vi "メイン.vi"() -> (2 "測定周期/ms":dbl, 3 "値転記用配列":T2[](array[typedef]))   [LabVIEW 2021] (continued)
                  tunnel: w3711 -> [w3725]
                  tunnel: [w3725] -> w3710
                  frame #0 {
                    w3720 = T9 {"Horizontal"=-51, "Vertical"=72} ("座標 2")
                    n1890 = control-ref of="このVI"() -> (w3724:refnum<vi>)
                    n1891 = property on="ペーン 2" class="Pane"("Origin"=w3720) -> ()  [unwired: 2 in, 2 out]
                    n1892 = property on="ペーン 2" class="Pane"("Origin"=w3720) -> ()  [unwired: 2 in, 2 out]
                    n1893 = control-ref of="このVI"() -> (w3722:refnum<vi>)
                    n1894 = Unbundle(w3720) -> ("Vertical"=w3723:i16)  [unwired: 1 out]
                    n1895 = Unbundle(w3720) -> ("Vertical"=w3721:i16)  [unwired: 1 out]
                    n1896 = call "メイン_装飾移動サブ.vi"("Y軸座標入力"=w3723, "VI入力"=w3724) -> ()  [unwired: 10 in]
                    n1897 = call "メイン_装飾枠移動サブ.vi"("Y軸座標入力"=w3721, "VI入力"=w3722) -> ()  [unwired: 10 in]
                  }
                }
              }
              frame #1 {
                w3955 = T8."Enabled" ("無効")
                # "⑪ボタンの無効解除"
                n1898 = local write "測定新値\nリセット用 2"(TRUE) -> ()
                n1899 = for {
                  N: 12 -> [_]
                  tunnel: w3955 -> [w3958]
                  i -> [w3959]
                  n1900 = case shown="11" w3959 {
                    tunnel: w3958 -> [w3960 w3961 w3962 w3963 w3964 w3965 w3966 w3967 w3968 w3969 w3970 w3971]
                    frame 0, Default {
                      n1901 = property on="メイン測定ボタン_単発 1" class="Bool (指定)"("DisabledEnum"=w3960) -> ()  [unwired: 2 in, 2 out]
                      n1902 = property on="メイン測定ボタン_連続 1" class="Bool (指定)"("DisabledEnum"=w3960) -> ()  [unwired: 2 in, 2 out]
                    }
                    frame 1 {
                      n1903 = property on="メイン測定ボタン_単発 2" class="Bool (指定)"("DisabledEnum"=w3961) -> ()  [unwired: 2 in, 2 out]
                      n1904 = property on="メイン測定ボタン_連続 2" class="Bool (指定)"("DisabledEnum"=w3961) -> ()  [unwired: 2 in, 2 out]
                    }
                    frame 2 {
                      n1905 = property on="メイン測定ボタン_単発 3" class="Bool (指定)"("DisabledEnum"=w3962) -> ()  [unwired: 2 in, 2 out]
                      n1906 = property on="メイン測定ボタン_連続 3" class="Bool (指定)"("DisabledEnum"=w3962) -> ()  [unwired: 2 in, 2 out]
                    }
                    frame 3 {
                      n1907 = property on="メイン測定ボタン_単発 4" class="Bool (指定)"("DisabledEnum"=w3963) -> ()  [unwired: 2 in, 2 out]
                      n1908 = property on="メイン測定ボタン_連続 4" class="Bool (指定)"("DisabledEnum"=w3963) -> ()  [unwired: 2 in, 2 out]
                    }
                    frame 4 {
                      n1909 = property on="メイン測定ボタン_単発 5" class="Bool (指定)"("DisabledEnum"=w3964) -> ()  [unwired: 2 in, 2 out]
                      n1910 = property on="メイン測定ボタン_連続 5" class="Bool (指定)"("DisabledEnum"=w3964) -> ()  [unwired: 2 in, 2 out]
                    }
                    frame 5 {
                      n1911 = property on="メイン測定ボタン_連続 6" class="Bool (指定)"("DisabledEnum"=w3965) -> ()  [unwired: 2 in, 2 out]
                      n1912 = property on="メイン測定ボタン_単発 6" class="Bool (指定)"("DisabledEnum"=w3965) -> ()  [unwired: 2 in, 2 out]
                    }
                    frame 6 {
                      n1913 = property on="メイン測定ボタン_連続 7" class="Bool (指定)"("DisabledEnum"=w3966) -> ()  [unwired: 2 in, 2 out]
                      n1914 = property on="メイン測定ボタン_単発 7" class="Bool (指定)"("DisabledEnum"=w3966) -> ()  [unwired: 2 in, 2 out]
                    }
                    frame 7 {
                      n1915 = property on="メイン測定ボタン_単発 8" class="Bool (指定)"("DisabledEnum"=w3967) -> ()  [unwired: 2 in, 2 out]
                      n1916 = property on="メイン測定ボタン_連続 8" class="Bool (指定)"("DisabledEnum"=w3967) -> ()  [unwired: 2 in, 2 out]
                    }
                    frame 8 {
                      n1917 = property on="メイン測定ボタン_単発 9" class="Bool (指定)"("DisabledEnum"=w3968) -> ()  [unwired: 2 in, 2 out]
                      n1918 = property on="メイン測定ボタン_連続 9" class="Bool (指定)"("DisabledEnum"=w3968) -> ()  [unwired: 2 in, 2 out]
                    }
                    frame 9 {
                      n1919 = property on="メイン測定ボタン_単発 10" class="Bool (指定)"("DisabledEnum"=w3969) -> ()  [unwired: 2 in, 2 out]
                      n1920 = property on="メイン測定ボタン_連続 10" class="Bool (指定)"("DisabledEnum"=w3969) -> ()  [unwired: 2 in, 2 out]
                    }
                    frame 10 {
                      n1921 = property on="メイン測定ボタン_単発 11" class="Bool (指定)"("DisabledEnum"=w3970) -> ()  [unwired: 2 in, 2 out]
                      n1922 = property on="メイン測定ボタン_連続 11" class="Bool (指定)"("DisabledEnum"=w3970) -> ()  [unwired: 2 in, 2 out]
                    }
                    frame 11 {
                      n1923 = property on="メイン測定ボタン_連続 12" class="Bool (指定)"("DisabledEnum"=w3971) -> ()  [unwired: 2 in, 2 out]
                      n1924 = property on="メイン測定ボタン_単発 12" class="Bool (指定)"("DisabledEnum"=w3971) -> ()  [unwired: 2 in, 2 out]
                    }
                  }
                }
                n1925 = property on="TOPページへ" class="Bool"("DisabledEnum"=w3955) -> ()  [unwired: 2 in, 2 out]
                n1926 = property on="保存して終了" class="Bool"("DisabledEnum"=w3955) -> ()  [unwired: 2 in, 2 out]
                n1927 = property on="保存せずに" class="Bool"("DisabledEnum"=w3955) -> ()  [unwired: 2 in, 2 out]
              }
            }
          }
          frame True {
          }
        }
      }
      frame "測定3" {
        # "⑦"
        # "項目別のボタンで測定を行う為、項目分必要"
        n1928 = local read "測定旧値 3"() -> (w3975:bool)
        n1929 = case shown="FALSE" w3975 {
          tunnel: w3973 -> [w3978 w4241]
          tunnel: [w3977 w4241] -> w3974
          frame False {
            n1930 = flat-sequence {
              tunnel: w3978 -> [w3988]
              tunnel: [w3980] -> w3976
              tunnel: [w4226] -> w3977
              tunnel: w3976 -> [w4226]
              frame #0 {
                # "※複製コピー時変更する項目\n①②\nローカル変数\n\n入れ子のケースストラクチャ\"2\"を複製\n\n0～数だけ変更する\n③④⑤\nローカル変数\n\n※AB\n行番号の変更をする必要がある\n\n--------------------------------\nこの後イベントストラクチャ複製する\n--------------------------------\nイベントストラクチャ複製後\n\n⑦⑧\nローカル変数\n⑨\n装飾体の位置設定\n-51は固定\n前ケースの数値+72\n⑩\n測定新値リセット用\nのボタンが複製されているので、\nフロントパネルを整理する\n⑪\nプロパティノード\nボタンの無効解除クリア以外全てのボタン対象"
                # "実測完了の簡易疑似コード\n\n1)測定モードが単発・連続、多点かで転記する配列を変える\n2)値転記用配列へ転記\n\nここからゲージ分を繰り返す必要がある\n\n3)配列0を取り出す\n4)配列0のポートNoを取り出す\n5)メイン測定_設定配列(測定1の対象配列)のポートNoと比較\n6)同じだったら処理をする。違ったら何もしない\n7)同じだったら配列0のメインON/OFF_設定1の使用ON/OFFがTrueかFalseか\nFlaseだったら前回値転記用配列から前回の値をメイン設定_設定へ転記\nTrueだったらメイン設定_設定の測定モードから\n0単発、1連続、3多点\nの処理を行う\n8)測定値をメイン設定_設定へ転記したら、前回転記用配列へ転記する"
                # "⑨"
                # "⑧"
                # "②"
                # "グループNO(表示上はポートNo)が同じだったら値を転記する\n\n測定した配列のグループNOと値転記用配列の他の指標グループNOを比較する\n＝だったら、対象の配列のON/OFFボタンがTrueか確認し、\nTrueだったら、測定モードによって、値かMAX、MINの数値を転記する\n\nグループNOが同じでなければ、転記しない(何もしない)"
                # "まず値転記用配列に測定の値を転記"
                # "実測定画面vi動作"
                n1931 = local read "メイン設定_設定 3"() -> (w3983:T2)
                n1932 = local read "測定新値 3"() -> (→"測定新値\nリセット用 3":bool)
                n1933 = local read "測定周期/ms"() -> (w3981:dbl)
                n1934 = Unbundle By Name(w3983) -> ("測定モード"=w3984:u16)
                n1935 = call "実測定画面.vi"("実測設定項目配列_\nメインからの転記"=w3988, "測定周期/ms_制御器"=w3981) -> ("実測設定項目配列_\nゲージIOへ転記用"=w3986:T2[], "実測設定項目配列_\n多点測定メイン転記用"=w3985:T2[])  [unwired: 11 in, 1 out]
                n1936 = case shown="1" w3984 {
                  tunnel: w3986 -> [w3995 w3996 _]
                  tunnel: [w3995 w3996 w3997] -> w3979
                  tunnel: w3985 -> [_ _ w3997]
                  frame 0, Default {
                  }
                  frame 1 {
                  }
                  frame 2 {
                  }
                }
                n1937 = for {
                  N: 32 -> [_]
                  tunnel: w3979 -> [w4004]
                  i -> [w3999]
                  # "①"
                  # "※複製コピーはこのケースで行う"
                  # "32回分"
                  # "比較する固定GNO"
                  n1938 = local read "メイン設定_設定 3"() -> (w3998:T2)
                  n1939 = Index Array(array=w4004, index=w3999) -> (element=w4003:T2)
                  n1940 = Unbundle By Name(w3998) -> ("ポートNo."=w4002:dbl)
                  n1941 = Unbundle By Name(w4003) -> ("ポートNo."=w4001:dbl)
                  n1942 = Equal?(x=w4002, y=w4001) -> (x = y?=w4000:bool)
                  n1943 = case shown="TRUE" w4000 {
                    tunnel: w4003 -> [_ w4006]
                    tunnel: w3999 -> [_ w4005]
                    frame False {
                    }
                    frame True {
                      n1944 = case shown="0, デフォルト" w4005 {
                        tunnel: w4006 -> [w4022 w4040 w4058 w4076 w4094 w4112 w4130 w4148 w4166 w4184 w4202 w4220]
                        tunnel: w4005 -> [w4021 w4039 w4057 w4075 w4093 w4111 w4129 w4147 w4165 w4183 w4201 w4219]
                        frame 0, Default {
                          w4012 = 2
                          # "B"
                          # "A"
                          # "csv作成の為表へクラスタ(実測値)書き込み"
                          # "⑤"
                          # "③"
                          # "④"
                          n1945 = local read "メインON/OFF_\n設定 1"() -> (w4023:T1)
                          n1946 = Unbundle By Name(w4023) -> ("使用ON/OFF"=w4019:bool)
                          n1947 = control-ref of="前回値転記用配列"() -> (w4017:refnum<vi>)
                          n1948 = local read "メイン設定_設定 1"() -> (w4024:T2)
                          n1949 = call "メイン_測定値配列_CSV転記サブ.vi"("メイン設定_設定入力"=w4024, "ループ反復数値入力"=w4021, "実測設定項目"=w4022, "使用ON/OFF"=w4019, "前回値転記用配列"=w4017) -> ("ループ反復数値出力"=w4020:i32, "メイン設定_設定出力"=w4018:T2)  [unwired: 5 in]
                          n1950 = local write "メイン設定_設定 1"(w4018) -> ()
                          n1951 = Add(x=2, y=w4020) -> (x+y=w4013:i32)
                          n1952 = Add(x=w4020, y=3) -> (x+y=w4011:i32)
                          n1953 = local read "csv作成表"() -> (w4007:string[][])
                          n1954 = Unbundle By Name(w4018) -> ("実測値(MAX)"=w4014:string, "実測値(MIN)"=w4015:string)
                          n1955 = Replace Array Subset(array=w4007, new element #1=w4014, index (row) #1=w4012, index (col) #1=w4013, new element #2=w4015, index (row) #2=w4012, index (col) #2=w4011) -> (w4009:string[][])
                          n1956 = Select(t=w4009, s=w4019, f=w4007) -> (s? t:f=w4010:string[][])
                          n1957 = local write "csv作成表"(w4010) -> ()
                        }
                        frame 1 {
                          w4030 = 2
                          # "B"
                          # "A"
                          # "csv作成の為表へクラスタ(実測値)書き込み"
                          # "⑤"
                          # "③"
                          # "④"
                          n1958 = local read "メインON/OFF_\n設定 2"() -> (w4041:T1)
                          n1959 = Unbundle By Name(w4041) -> ("使用ON/OFF"=w4037:bool)
                          n1960 = control-ref of="前回値転記用配列"() -> (w4035:refnum<vi>)
                          n1961 = local read "メイン設定_設定 2"() -> (w4042:T2)
                          n1962 = call "メイン_測定値配列_CSV転記サブ.vi"("メイン設定_設定入力"=w4042, "ループ反復数値入力"=w4039, "実測設定項目"=w4040, "使用ON/OFF"=w4037, "前回値転記用配列"=w4035) -> ("ループ反復数値出力"=w4038:i32, "メイン設定_設定出力"=w4036:T2)  [unwired: 5 in]
                          n1963 = local write "メイン設定_設定 2"(w4036) -> ()
                          n1964 = Add(x=3, y=w4038) -> (x+y=w4031:i32)
                          n1965 = Add(x=w4038, y=4) -> (x+y=w4029:i32)
                          n1966 = local read "csv作成表"() -> (w4025:string[][])
                          n1967 = Unbundle By Name(w4036) -> ("実測値(MAX)"=w4032:string, "実測値(MIN)"=w4033:string)
                          n1968 = Replace Array Subset(array=w4025, new element #1=w4032, index (row) #1=w4030, index (col) #1=w4031, new element #2=w4033, index (row) #2=w4030, index (col) #2=w4029) -> (w4027:string[][])
                          n1969 = Select(t=w4027, s=w4037, f=w4025) -> (s? t:f=w4028:string[][])
                          n1970 = local write "csv作成表"(w4028) -> ()
                        }
                        frame 2 {
                          w4048 = 2
                          # "B"
                          # "A"
                          # "csv作成の為表へクラスタ(実測値)書き込み"
                          # "⑤"
                          # "③"
                          # "④"
                          n1971 = local read "メインON/OFF_\n設定 3"() -> (w4059:T1)
                          n1972 = Unbundle By Name(w4059) -> ("使用ON/OFF"=w4055:bool)
                          n1973 = control-ref of="前回値転記用配列"() -> (w4053:refnum<vi>)
                          n1974 = local read "メイン設定_設定 3"() -> (w4060:T2)
                          n1975 = call "メイン_測定値配列_CSV転記サブ.vi"("メイン設定_設定入力"=w4060, "ループ反復数値入力"=w4057, "実測設定項目"=w4058, "使用ON/OFF"=w4055, "前回値転記用配列"=w4053) -> ("ループ反復数値出力"=w4056:i32, "メイン設定_設定出力"=w4054:T2)  [unwired: 5 in]
                          n1976 = local write "メイン設定_設定 3"(w4054) -> ()
                          n1977 = Add(x=4, y=w4056) -> (x+y=w4049:i32)
                          n1978 = Add(x=w4056, y=5) -> (x+y=w4047:i32)
                          n1979 = local read "csv作成表"() -> (w4043:string[][])
                          n1980 = Unbundle By Name(w4054) -> ("実測値(MAX)"=w4050:string, "実測値(MIN)"=w4051:string)
                          n1981 = Replace Array Subset(array=w4043, new element #1=w4050, index (row) #1=w4048, index (col) #1=w4049, new element #2=w4051, index (row) #2=w4048, index (col) #2=w4047) -> (w4045:string[][])
                          n1982 = Select(t=w4045, s=w4055, f=w4043) -> (s? t:f=w4046:string[][])
                          n1983 = local write "csv作成表"(w4046) -> ()
                        }
                        frame 3 {
                          w4066 = 2
                          # "B"
                          # "A"
                          # "csv作成の為表へクラスタ(実測値)書き込み"
                          # "⑤"
                          # "③"
                          # "④"
                          n1984 = local read "メインON/OFF_\n設定 4"() -> (w4077:T1)
                          n1985 = Unbundle By Name(w4077) -> ("使用ON/OFF"=w4073:bool)
                          n1986 = control-ref of="前回値転記用配列"() -> (w4071:refnum<vi>)
                          n1987 = local read "メイン設定_設定 4"() -> (w4078:T2)
                          n1988 = call "メイン_測定値配列_CSV転記サブ.vi"("メイン設定_設定入力"=w4078, "ループ反復数値入力"=w4075, "実測設定項目"=w4076, "使用ON/OFF"=w4073, "前回値転記用配列"=w4071) -> ("ループ反復数値出力"=w4074:i32, "メイン設定_設定出力"=w4072:T2)  [unwired: 5 in]
                          n1989 = local write "メイン設定_設定 4"(w4072) -> ()
                          n1990 = Add(x=5, y=w4074) -> (x+y=w4067:i32)
                          n1991 = Add(x=w4074, y=6) -> (x+y=w4065:i32)
                          n1992 = local read "csv作成表"() -> (w4061:string[][])
                          n1993 = Unbundle By Name(w4072) -> ("実測値(MAX)"=w4068:string, "実測値(MIN)"=w4069:string)
                          n1994 = Replace Array Subset(array=w4061, new element #1=w4068, index (row) #1=w4066, index (col) #1=w4067, new element #2=w4069, index (row) #2=w4066, index (col) #2=w4065) -> (w4063:string[][])
                          n1995 = Select(t=w4063, s=w4073, f=w4061) -> (s? t:f=w4064:string[][])
                          n1996 = local write "csv作成表"(w4064) -> ()
                        }
                        frame 4 {
                          w4084 = 2
                          # "B"
                          # "A"
                          # "csv作成の為表へクラスタ(実測値)書き込み"
                          # "⑤"
                          # "③"
                          # "④"
                          n1997 = local read "メインON/OFF_\n設定 5"() -> (w4095:T1)
                          n1998 = Unbundle By Name(w4095) -> ("使用ON/OFF"=w4091:bool)
                          n1999 = control-ref of="前回値転記用配列"() -> (w4089:refnum<vi>)
                          n2000 = local read "メイン設定_設定 5"() -> (w4096:T2)
                          n2001 = call "メイン_測定値配列_CSV転記サブ.vi"("メイン設定_設定入力"=w4096, "ループ反復数値入力"=w4093, "実測設定項目"=w4094, "使用ON/OFF"=w4091, "前回値転記用配列"=w4089) -> ("ループ反復数値出力"=w4092:i32, "メイン設定_設定出力"=w4090:T2)  [unwired: 5 in]
                          n2002 = local write "メイン設定_設定 5"(w4090) -> ()
                          n2003 = Add(x=6, y=w4092) -> (x+y=w4085:i32)
                          n2004 = Add(x=w4092, y=7) -> (x+y=w4083:i32)
                          n2005 = local read "csv作成表"() -> (w4079:string[][])
                          n2006 = Unbundle By Name(w4090) -> ("実測値(MAX)"=w4086:string, "実測値(MIN)"=w4087:string)
                          n2007 = Replace Array Subset(array=w4079, new element #1=w4086, index (row) #1=w4084, index (col) #1=w4085, new element #2=w4087, index (row) #2=w4084, index (col) #2=w4083) -> (w4081:string[][])
                          n2008 = Select(t=w4081, s=w4091, f=w4079) -> (s? t:f=w4082:string[][])
                          n2009 = local write "csv作成表"(w4082) -> ()
                        }
                        frame 5 {
                          w4102 = 2
                          # "B"
                          # "A"
                          # "csv作成の為表へクラスタ(実測値)書き込み"
                          # "⑤"
                          # "③"
                          # "④"
                          n2010 = local read "メインON/OFF_\n設定 6"() -> (w4113:T1)
                          n2011 = Unbundle By Name(w4113) -> ("使用ON/OFF"=w4109:bool)
                          n2012 = control-ref of="前回値転記用配列"() -> (w4107:refnum<vi>)
                          n2013 = local read "メイン設定_設定 6"() -> (w4114:T2)
                          n2014 = call "メイン_測定値配列_CSV転記サブ.vi"("メイン設定_設定入力"=w4114, "ループ反復数値入力"=w4111, "実測設定項目"=w4112, "使用ON/OFF"=w4109, "前回値転記用配列"=w4107) -> ("ループ反復数値出力"=w4110:i32, "メイン設定_設定出力"=w4108:T2)  [unwired: 5 in]
                          n2015 = local write "メイン設定_設定 6"(w4108) -> ()
                          n2016 = Add(x=7, y=w4110) -> (x+y=w4103:i32)
                          n2017 = Add(x=w4110, y=8) -> (x+y=w4101:i32)
                          n2018 = local read "csv作成表"() -> (w4097:string[][])
                          n2019 = Unbundle By Name(w4108) -> ("実測値(MAX)"=w4104:string, "実測値(MIN)"=w4105:string)
                          n2020 = Replace Array Subset(array=w4097, new element #1=w4104, index (row) #1=w4102, index (col) #1=w4103, new element #2=w4105, index (row) #2=w4102, index (col) #2=w4101) -> (w4099:string[][])
                          n2021 = Select(t=w4099, s=w4109, f=w4097) -> (s? t:f=w4100:string[][])
                          n2022 = local write "csv作成表"(w4100) -> ()
                        }
                        frame 6 {
                          w4120 = 2
                          # "B"
                          # "A"
                          # "csv作成の為表へクラスタ(実測値)書き込み"
                          # "⑤"
                          # "③"
                          # "④"
                          n2023 = local read "メインON/OFF_\n設定 7"() -> (w4131:T1)
                          n2024 = Unbundle By Name(w4131) -> ("使用ON/OFF"=w4127:bool)
                          n2025 = control-ref of="前回値転記用配列"() -> (w4125:refnum<vi>)
                          n2026 = local read "メイン設定_設定 7"() -> (w4132:T2)
                          n2027 = call "メイン_測定値配列_CSV転記サブ.vi"("メイン設定_設定入力"=w4132, "ループ反復数値入力"=w4129, "実測設定項目"=w4130, "使用ON/OFF"=w4127, "前回値転記用配列"=w4125) -> ("ループ反復数値出力"=w4128:i32, "メイン設定_設定出力"=w4126:T2)  [unwired: 5 in]
                          n2028 = local write "メイン設定_設定 7"(w4126) -> ()
                          n2029 = Add(x=8, y=w4128) -> (x+y=w4121:i32)
                          n2030 = Add(x=w4128, y=9) -> (x+y=w4119:i32)
                          n2031 = local read "csv作成表"() -> (w4115:string[][])
                          n2032 = Unbundle By Name(w4126) -> ("実測値(MAX)"=w4122:string, "実測値(MIN)"=w4123:string)
                          n2033 = Replace Array Subset(array=w4115, new element #1=w4122, index (row) #1=w4120, index (col) #1=w4121, new element #2=w4123, index (row) #2=w4120, index (col) #2=w4119) -> (w4117:string[][])
                          n2034 = Select(t=w4117, s=w4127, f=w4115) -> (s? t:f=w4118:string[][])
                          n2035 = local write "csv作成表"(w4118) -> ()
                        }
                        frame 7 {
                          w4138 = 2
                          # "B"
                          # "A"
                          # "csv作成の為表へクラスタ(実測値)書き込み"
                          # "⑤"
                          # "③"
                          # "④"
                          n2036 = local read "メインON/OFF_\n設定 8"() -> (w4149:T1)
                          n2037 = Unbundle By Name(w4149) -> ("使用ON/OFF"=w4145:bool)
                          n2038 = control-ref of="前回値転記用配列"() -> (w4143:refnum<vi>)
                          n2039 = local read "メイン設定_設定 8"() -> (w4150:T2)
                          n2040 = call "メイン_測定値配列_CSV転記サブ.vi"("メイン設定_設定入力"=w4150, "ループ反復数値入力"=w4147, "実測設定項目"=w4148, "使用ON/OFF"=w4145, "前回値転記用配列"=w4143) -> ("ループ反復数値出力"=w4146:i32, "メイン設定_設定出力"=w4144:T2)  [unwired: 5 in]
                          n2041 = local write "メイン設定_設定 8"(w4144) -> ()
                          n2042 = Add(x=9, y=w4146) -> (x+y=w4139:i32)
                          n2043 = Add(x=w4146, y=10) -> (x+y=w4137:i32)
                          n2044 = local read "csv作成表"() -> (w4133:string[][])
                          n2045 = Unbundle By Name(w4144) -> ("実測値(MAX)"=w4140:string, "実測値(MIN)"=w4141:string)
                          n2046 = Replace Array Subset(array=w4133, new element #1=w4140, index (row) #1=w4138, index (col) #1=w4139, new element #2=w4141, index (row) #2=w4138, index (col) #2=w4137) -> (w4135:string[][])
                          n2047 = Select(t=w4135, s=w4145, f=w4133) -> (s? t:f=w4136:string[][])
                          n2048 = local write "csv作成表"(w4136) -> ()
                        }
                        frame 8 {
                          w4156 = 2
                          # "B"
                          # "A"
                          # "csv作成の為表へクラスタ(実測値)書き込み"
                          # "⑤"
                          # "③"
                          # "④"
                          n2049 = local read "メインON/OFF_\n設定 9"() -> (w4167:T1)
                          n2050 = Unbundle By Name(w4167) -> ("使用ON/OFF"=w4163:bool)
                          n2051 = control-ref of="前回値転記用配列"() -> (w4161:refnum<vi>)
                          n2052 = local read "メイン設定_設定 9"() -> (w4168:T2)
                          n2053 = call "メイン_測定値配列_CSV転記サブ.vi"("メイン設定_設定入力"=w4168, "ループ反復数値入力"=w4165, "実測設定項目"=w4166, "使用ON/OFF"=w4163, "前回値転記用配列"=w4161) -> ("ループ反復数値出力"=w4164:i32, "メイン設定_設定出力"=w4162:T2)  [unwired: 5 in]
                          n2054 = local write "メイン設定_設定 9"(w4162) -> ()
                          n2055 = Add(x=10, y=w4164) -> (x+y=w4157:i32)
                          n2056 = Add(x=w4164, y=11) -> (x+y=w4155:i32)
                          n2057 = local read "csv作成表"() -> (w4151:string[][])
                          n2058 = Unbundle By Name(w4162) -> ("実測値(MAX)"=w4158:string, "実測値(MIN)"=w4159:string)
                          n2059 = Replace Array Subset(array=w4151, new element #1=w4158, index (row) #1=w4156, index (col) #1=w4157, new element #2=w4159, index (row) #2=w4156, index (col) #2=w4155) -> (w4153:string[][])
                          n2060 = Select(t=w4153, s=w4163, f=w4151) -> (s? t:f=w4154:string[][])
                          n2061 = local write "csv作成表"(w4154) -> ()
                        }
                        frame 9 {
                          w4174 = 2
                          # "B"
                          # "A"
                          # "csv作成の為表へクラスタ(実測値)書き込み"
                          # "⑤"
                          # "③"
                          # "④"
                          n2062 = local read "メインON/OFF_\n設定 10"() -> (w4185:T1)
                          n2063 = Unbundle By Name(w4185) -> ("使用ON/OFF"=w4181:bool)
                          n2064 = control-ref of="前回値転記用配列"() -> (w4179:refnum<vi>)
                          n2065 = local read "メイン設定_設定 10"() -> (w4186:T2)
                          n2066 = call "メイン_測定値配列_CSV転記サブ.vi"("メイン設定_設定入力"=w4186, "ループ反復数値入力"=w4183, "実測設定項目"=w4184, "使用ON/OFF"=w4181, "前回値転記用配列"=w4179) -> ("ループ反復数値出力"=w4182:i32, "メイン設定_設定出力"=w4180:T2)  [unwired: 5 in]
                          n2067 = local write "メイン設定_設定 10"(w4180) -> ()
                          n2068 = Add(x=11, y=w4182) -> (x+y=w4175:i32)
                          n2069 = Add(x=w4182, y=12) -> (x+y=w4173:i32)
                          n2070 = local read "csv作成表"() -> (w4169:string[][])
                          n2071 = Unbundle By Name(w4180) -> ("実測値(MAX)"=w4176:string, "実測値(MIN)"=w4177:string)
                          n2072 = Replace Array Subset(array=w4169, new element #1=w4176, index (row) #1=w4174, index (col) #1=w4175, new element #2=w4177, index (row) #2=w4174, index (col) #2=w4173) -> (w4171:string[][])
                          n2073 = Select(t=w4171, s=w4181, f=w4169) -> (s? t:f=w4172:string[][])
                          n2074 = local write "csv作成表"(w4172) -> ()
                        }
                        frame 10 {
                          w4192 = 2
                          # "B"
                          # "A"
                          # "csv作成の為表へクラスタ(実測値)書き込み"
                          # "⑤"
                          # "③"
                          # "④"
                          n2075 = local read "メインON/OFF_\n設定 11"() -> (w4203:T1)
                          n2076 = Unbundle By Name(w4203) -> ("使用ON/OFF"=w4199:bool)
                          n2077 = control-ref of="前回値転記用配列"() -> (w4197:refnum<vi>)
                          n2078 = local read "メイン設定_設定 11"() -> (w4204:T2)
                          n2079 = call "メイン_測定値配列_CSV転記サブ.vi"("メイン設定_設定入力"=w4204, "ループ反復数値入力"=w4201, "実測設定項目"=w4202, "使用ON/OFF"=w4199, "前回値転記用配列"=w4197) -> ("ループ反復数値出力"=w4200:i32, "メイン設定_設定出力"=w4198:T2)  [unwired: 5 in]
                          n2080 = local write "メイン設定_設定 11"(w4198) -> ()
                          n2081 = Add(x=12, y=w4200) -> (x+y=w4193:i32)
                          n2082 = Add(x=w4200, y=13) -> (x+y=w4191:i32)
                          n2083 = local read "csv作成表"() -> (w4187:string[][])
                          n2084 = Unbundle By Name(w4198) -> ("実測値(MAX)"=w4194:string, "実測値(MIN)"=w4195:string)
                          n2085 = Replace Array Subset(array=w4187, new element #1=w4194, index (row) #1=w4192, index (col) #1=w4193, new element #2=w4195, index (row) #2=w4192, index (col) #2=w4191) -> (w4189:string[][])
                          n2086 = Select(t=w4189, s=w4199, f=w4187) -> (s? t:f=w4190:string[][])
                          n2087 = local write "csv作成表"(w4190) -> ()
                        }
                        frame 11 {
                          w4210 = 2
                          # "B"
                          # "A"
                          # "csv作成の為表へクラスタ(実測値)書き込み"
                          # "⑤"
                          # "③"
                          # "④"
                          n2088 = local read "メインON/OFF_\n設定 12"() -> (w4221:T1)
                          n2089 = Unbundle By Name(w4221) -> ("使用ON/OFF"=w4217:bool)
                          n2090 = control-ref of="前回値転記用配列"() -> (w4215:refnum<vi>)
                          n2091 = local read "メイン設定_設定 12"() -> (w4222:T2)
                          n2092 = call "メイン_測定値配列_CSV転記サブ.vi"("メイン設定_設定入力"=w4222, "ループ反復数値入力"=w4219, "実測設定項目"=w4220, "使用ON/OFF"=w4217, "前回値転記用配列"=w4215) -> ("ループ反復数値出力"=w4218:i32, "メイン設定_設定出力"=w4216:T2)  [unwired: 5 in]
                          n2093 = local write "メイン設定_設定 12"(w4216) -> ()
                          n2094 = Add(x=13, y=w4218) -> (x+y=w4211:i32)
                          n2095 = Add(x=w4218, y=14) -> (x+y=w4209:i32)
                          n2096 = local read "csv作成表"() -> (w4205:string[][])
                          n2097 = Unbundle By Name(w4216) -> ("実測値(MAX)"=w4212:string, "実測値(MIN)"=w4213:string)
                          n2098 = Replace Array Subset(array=w4205, new element #1=w4212, index (row) #1=w4210, index (col) #1=w4211, new element #2=w4213, index (row) #2=w4210, index (col) #2=w4209) -> (w4207:string[][])
                          n2099 = Select(t=w4207, s=w4217, f=w4205) -> (s? t:f=w4208:string[][])
                          n2100 = local write "csv作成表"(w4208) -> ()
                        }
                      }
                    }
                  }
                }
                n2101 = local write "値転記用配列"(w3979) -> ()
                n2102 = flat-sequence {
                  tunnel: [w3994] -> w3980
                  tunnel: w3979 -> [w3994]
                  frame #0 {
                    w3989 = T9 {"Horizontal"=-51, "Vertical"=144} ("座標 2")
                    n2103 = control-ref of="このVI"() -> (w3990:refnum<vi>)
                    n2104 = property on="ペーン 2" class="Pane"("Origin"=w3989) -> ()  [unwired: 2 in, 2 out]
                    n2105 = property on="ペーン 2" class="Pane"("Origin"=w3989) -> ()  [unwired: 2 in, 2 out]
                    n2106 = control-ref of="このVI"() -> (w3992:refnum<vi>)
                    n2107 = Unbundle(w3989) -> ("Vertical"=w3991:i16)  [unwired: 1 out]
                    n2108 = Unbundle(w3989) -> ("Vertical"=w3993:i16)  [unwired: 1 out]
                    n2109 = call "メイン_装飾移動サブ.vi"("Y軸座標入力"=w3991, "VI入力"=w3990) -> ()  [unwired: 10 in]
                    n2110 = call "メイン_装飾枠移動サブ.vi"("Y軸座標入力"=w3993, "VI入力"=w3992) -> ()  [unwired: 10 in]
                  }
                }
              }
              frame #1 {
                w4224 = T8."Enabled" ("無効")
                # "⑪ボタンの無効解除"
                n2111 = for {
                  N: 12 -> [_]
                  tunnel: w4224 -> [w4227]
                  i -> [w4228]
                  n2112 = case shown="11" w4228 {
                    tunnel: w4227 -> [w4229 w4230 w4231 w4232 w4233 w4234 w4235 w4236 w4237 w4238 w4239 w4240]
                    frame 0, Default {
                      n2113 = property on="メイン測定ボタン_単発 1" class="Bool (指定)"("DisabledEnum"=w4229) -> ()  [unwired: 2 in, 2 out]
                      n2114 = property on="メイン測定ボタン_連続 1" class="Bool (指定)"("DisabledEnum"=w4229) -> ()  [unwired: 2 in, 2 out]
                    }
                    frame 1 {
                      n2115 = property on="メイン測定ボタン_単発 2" class="Bool (指定)"("DisabledEnum"=w4230) -> ()  [unwired: 2 in, 2 out]
                      n2116 = property on="メイン測定ボタン_連続 2" class="Bool (指定)"("DisabledEnum"=w4230) -> ()  [unwired: 2 in, 2 out]
                    }
                    frame 2 {
                      n2117 = property on="メイン測定ボタン_単発 3" class="Bool (指定)"("DisabledEnum"=w4231) -> ()  [unwired: 2 in, 2 out]
                      n2118 = property on="メイン測定ボタン_連続 3" class="Bool (指定)"("DisabledEnum"=w4231) -> ()  [unwired: 2 in, 2 out]
                    }
                    frame 3 {
                      n2119 = property on="メイン測定ボタン_単発 4" class="Bool (指定)"("DisabledEnum"=w4232) -> ()  [unwired: 2 in, 2 out]
                      n2120 = property on="メイン測定ボタン_連続 4" class="Bool (指定)"("DisabledEnum"=w4232) -> ()  [unwired: 2 in, 2 out]
                    }
                    frame 4 {
                      n2121 = property on="メイン測定ボタン_単発 5" class="Bool (指定)"("DisabledEnum"=w4233) -> ()  [unwired: 2 in, 2 out]
                      n2122 = property on="メイン測定ボタン_連続 5" class="Bool (指定)"("DisabledEnum"=w4233) -> ()  [unwired: 2 in, 2 out]
                    }
                    frame 5 {
                      n2123 = property on="メイン測定ボタン_連続 6" class="Bool (指定)"("DisabledEnum"=w4234) -> ()  [unwired: 2 in, 2 out]
                      n2124 = property on="メイン測定ボタン_単発 6" class="Bool (指定)"("DisabledEnum"=w4234) -> ()  [unwired: 2 in, 2 out]
                    }
                    frame 6 {
                      n2125 = property on="メイン測定ボタン_連続 7" class="Bool (指定)"("DisabledEnum"=w4235) -> ()  [unwired: 2 in, 2 out]
                      n2126 = property on="メイン測定ボタン_単発 7" class="Bool (指定)"("DisabledEnum"=w4235) -> ()  [unwired: 2 in, 2 out]
                    }
                    frame 7 {
                      n2127 = property on="メイン測定ボタン_単発 8" class="Bool (指定)"("DisabledEnum"=w4236) -> ()  [unwired: 2 in, 2 out]
                      n2128 = property on="メイン測定ボタン_連続 8" class="Bool (指定)"("DisabledEnum"=w4236) -> ()  [unwired: 2 in, 2 out]
                    }
                    frame 8 {
                      n2129 = property on="メイン測定ボタン_単発 9" class="Bool (指定)"("DisabledEnum"=w4237) -> ()  [unwired: 2 in, 2 out]
                      n2130 = property on="メイン測定ボタン_連続 9" class="Bool (指定)"("DisabledEnum"=w4237) -> ()  [unwired: 2 in, 2 out]
                    }
                    frame 9 {
                      n2131 = property on="メイン測定ボタン_単発 10" class="Bool (指定)"("DisabledEnum"=w4238) -> ()  [unwired: 2 in, 2 out]
                      n2132 = property on="メイン測定ボタン_連続 10" class="Bool (指定)"("DisabledEnum"=w4238) -> ()  [unwired: 2 in, 2 out]
                    }
                    frame 10 {
                      n2133 = property on="メイン測定ボタン_単発 11" class="Bool (指定)"("DisabledEnum"=w4239) -> ()  [unwired: 2 in, 2 out]
                      n2134 = property on="メイン測定ボタン_連続 11" class="Bool (指定)"("DisabledEnum"=w4239) -> ()  [unwired: 2 in, 2 out]
                    }
                    frame 11 {
                      n2135 = property on="メイン測定ボタン_連続 12" class="Bool (指定)"("DisabledEnum"=w4240) -> ()  [unwired: 2 in, 2 out]
                      n2136 = property on="メイン測定ボタン_単発 12" class="Bool (指定)"("DisabledEnum"=w4240) -> ()  [unwired: 2 in, 2 out]
                    }
                  }
                }
                n2137 = local write "測定新値\nリセット用 3"(TRUE) -> ()
                n2138 = property on="TOPページへ" class="Bool"("DisabledEnum"=w4224) -> ()  [unwired: 2 in, 2 out]
                n2139 = property on="保存して終了" class="Bool"("DisabledEnum"=w4224) -> ()  [unwired: 2 in, 2 out]
                n2140 = property on="保存せずに" class="Bool"("DisabledEnum"=w4224) -> ()  [unwired: 2 in, 2 out]
              }
            }
          }
          frame True {
          }
        }
      }
      frame "測定4" {
        # "⑦"
        # "項目別のボタンで測定を行う為、項目分必要"
        n2141 = local read "測定旧値 4"() -> (w4244:bool)
        n2142 = case shown="FALSE" w4244 {
          tunnel: w4242 -> [w4247 w4510]
          tunnel: [w4246 w4510] -> w4243
          frame False {
            n2143 = flat-sequence {
              tunnel: w4247 -> [w4257]
              tunnel: [w4249] -> w4245
              tunnel: [w4495] -> w4246
              tunnel: w4245 -> [w4495]
              frame #0 {
                # "※複製コピー時変更する項目\n①②\nローカル変数\n\n入れ子のケースストラクチャ\"2\"を複製\n\n0～数だけ変更する\n③④⑤\nローカル変数\n\n※AB\n行番号の変更をする必要がある\n\n--------------------------------\nこの後イベントストラクチャ複製する\n--------------------------------\nイベントストラクチャ複製後\n\n⑦⑧\nローカル変数\n⑨\n装飾体の位置設定\n-51は固定\n前ケースの数値+72\n⑩\n測定新値リセット用\nのボタンが複製されているので、\nフロントパネルを整理する\n⑪\nプロパティノード\nボタンの無効解除クリア以外全てのボタン対象"
                # "実測完了の簡易疑似コード\n\n1)測定モードが単発・連続、多点かで転記する配列を変える\n2)値転記用配列へ転記\n\nここからゲージ分を繰り返す必要がある\n\n3)配列0を取り出す\n4)配列0のポートNoを取り出す\n5)メイン測定_設定配列(測定1の対象配列)のポートNoと比較\n6)同じだったら処理をする。違ったら何もしない\n7)同じだったら配列0のメインON/OFF_設定1の使用ON/OFFがTrueかFalseか\nFlaseだったら前回値転記用配列から前回の値をメイン設定_設定へ転記\nTrueだったらメイン設定_設定の測定モードから\n0単発、1連続、3多点\nの処理を行う\n8)測定値をメイン設定_設定へ転記したら、前回転記用配列へ転記する"
                # "⑨"
                # "⑧"
                # "②"
                # "グループNO(表示上はポートNo)が同じだったら値を転記する\n\n測定した配列のグループNOと値転記用配列の他の指標グループNOを比較する\n＝だったら、対象の配列のON/OFFボタンがTrueか確認し、\nTrueだったら、測定モードによって、値かMAX、MINの数値を転記する\n\nグループNOが同じでなければ、転記しない(何もしない)"
                # "まず値転記用配列に測定の値を転記"
                # "実測定画面vi動作"
                n2144 = local read "メイン設定_設定 4"() -> (w4252:T2)
                n2145 = local read "測定新値 4"() -> (→"測定新値\nリセット用 4":bool)
                n2146 = local read "測定周期/ms"() -> (w4250:dbl)
                n2147 = Unbundle By Name(w4252) -> ("測定モード"=w4253:u16)
                n2148 = call "実測定画面.vi"("実測設定項目配列_\nメインからの転記"=w4257, "測定周期/ms_制御器"=w4250) -> ("実測設定項目配列_\nゲージIOへ転記用"=w4255:T2[], "実測設定項目配列_\n多点測定メイン転記用"=w4254:T2[])  [unwired: 11 in, 1 out]
                n2149 = case shown="1" w4253 {
                  tunnel: w4255 -> [w4264 w4265 _]
                  tunnel: [w4264 w4265 w4266] -> w4248
                  tunnel: w4254 -> [_ _ w4266]
                  frame 0, Default {
                  }
                  frame 1 {
                  }
                  frame 2 {
                  }
                }
                n2150 = for {
                  N: 32 -> [_]
                  tunnel: w4248 -> [w4273]
                  i -> [w4268]
                  # "①"
                  # "※複製コピーはこのケースで行う"
                  # "32回分"
                  # "比較する固定GNO"
                  n2151 = local read "メイン設定_設定 4"() -> (w4267:T2)
                  n2152 = Index Array(array=w4273, index=w4268) -> (element=w4272:T2)
                  n2153 = Unbundle By Name(w4267) -> ("ポートNo."=w4271:dbl)
                  n2154 = Unbundle By Name(w4272) -> ("ポートNo."=w4270:dbl)
                  n2155 = Equal?(x=w4271, y=w4270) -> (x = y?=w4269:bool)
                  n2156 = case shown="TRUE" w4269 {
                    tunnel: w4272 -> [_ w4275]
                    tunnel: w4268 -> [_ w4274]
                    frame False {
                    }
                    frame True {
                      n2157 = case shown="0, デフォルト" w4274 {
                        tunnel: w4275 -> [w4291 w4309 w4327 w4345 w4363 w4381 w4399 w4417 w4435 w4453 w4471 w4489]
                        tunnel: w4274 -> [w4290 w4308 w4326 w4344 w4362 w4380 w4398 w4416 w4434 w4452 w4470 w4488]
                        frame 0, Default {
                          w4281 = 2
                          # "B"
                          # "A"
                          # "csv作成の為表へクラスタ(実測値)書き込み"
                          # "⑤"
                          # "③"
                          # "④"
                          n2158 = local read "メインON/OFF_\n設定 1"() -> (w4292:T1)
                          n2159 = Unbundle By Name(w4292) -> ("使用ON/OFF"=w4288:bool)
                          n2160 = control-ref of="前回値転記用配列"() -> (w4286:refnum<vi>)
                          n2161 = local read "メイン設定_設定 1"() -> (w4293:T2)
                          n2162 = call "メイン_測定値配列_CSV転記サブ.vi"("メイン設定_設定入力"=w4293, "ループ反復数値入力"=w4290, "実測設定項目"=w4291, "使用ON/OFF"=w4288, "前回値転記用配列"=w4286) -> ("ループ反復数値出力"=w4289:i32, "メイン設定_設定出力"=w4287:T2)  [unwired: 5 in]
                          n2163 = local write "メイン設定_設定 1"(w4287) -> ()
                          n2164 = Add(x=2, y=w4289) -> (x+y=w4282:i32)
                          n2165 = Add(x=w4289, y=3) -> (x+y=w4280:i32)
                          n2166 = local read "csv作成表"() -> (w4276:string[][])
                          n2167 = Unbundle By Name(w4287) -> ("実測値(MAX)"=w4283:string, "実測値(MIN)"=w4284:string)
                          n2168 = Replace Array Subset(array=w4276, new element #1=w4283, index (row) #1=w4281, index (col) #1=w4282, new element #2=w4284, index (row) #2=w4281, index (col) #2=w4280) -> (w4278:string[][])
                          n2169 = Select(t=w4278, s=w4288, f=w4276) -> (s? t:f=w4279:string[][])
                          n2170 = local write "csv作成表"(w4279) -> ()
                        }
                        frame 1 {
                          w4299 = 2
                          # "B"
                          # "A"
                          # "csv作成の為表へクラスタ(実測値)書き込み"
                          # "⑤"
                          # "③"
                          # "④"
                          n2171 = local read "メインON/OFF_\n設定 2"() -> (w4310:T1)
                          n2172 = Unbundle By Name(w4310) -> ("使用ON/OFF"=w4306:bool)
                          n2173 = control-ref of="前回値転記用配列"() -> (w4304:refnum<vi>)
                          n2174 = local read "メイン設定_設定 2"() -> (w4311:T2)
                          n2175 = call "メイン_測定値配列_CSV転記サブ.vi"("メイン設定_設定入力"=w4311, "ループ反復数値入力"=w4308, "実測設定項目"=w4309, "使用ON/OFF"=w4306, "前回値転記用配列"=w4304) -> ("ループ反復数値出力"=w4307:i32, "メイン設定_設定出力"=w4305:T2)  [unwired: 5 in]
                          n2176 = local write "メイン設定_設定 2"(w4305) -> ()
                          n2177 = Add(x=3, y=w4307) -> (x+y=w4300:i32)
                          n2178 = Add(x=w4307, y=4) -> (x+y=w4298:i32)
                          n2179 = local read "csv作成表"() -> (w4294:string[][])
                          n2180 = Unbundle By Name(w4305) -> ("実測値(MAX)"=w4301:string, "実測値(MIN)"=w4302:string)
                          n2181 = Replace Array Subset(array=w4294, new element #1=w4301, index (row) #1=w4299, index (col) #1=w4300, new element #2=w4302, index (row) #2=w4299, index (col) #2=w4298) -> (w4296:string[][])
                          n2182 = Select(t=w4296, s=w4306, f=w4294) -> (s? t:f=w4297:string[][])
                          n2183 = local write "csv作成表"(w4297) -> ()
                        }
                        frame 2 {
                          w4317 = 2
                          # "B"
                          # "A"
                          # "csv作成の為表へクラスタ(実測値)書き込み"
                          # "⑤"
                          # "③"
                          # "④"
                          n2184 = local read "メインON/OFF_\n設定 3"() -> (w4328:T1)
                          n2185 = Unbundle By Name(w4328) -> ("使用ON/OFF"=w4324:bool)
                          n2186 = control-ref of="前回値転記用配列"() -> (w4322:refnum<vi>)
                          n2187 = local read "メイン設定_設定 3"() -> (w4329:T2)
                          n2188 = call "メイン_測定値配列_CSV転記サブ.vi"("メイン設定_設定入力"=w4329, "ループ反復数値入力"=w4326, "実測設定項目"=w4327, "使用ON/OFF"=w4324, "前回値転記用配列"=w4322) -> ("ループ反復数値出力"=w4325:i32, "メイン設定_設定出力"=w4323:T2)  [unwired: 5 in]
                          n2189 = local write "メイン設定_設定 3"(w4323) -> ()
                          n2190 = Add(x=4, y=w4325) -> (x+y=w4318:i32)
                          n2191 = Add(x=w4325, y=5) -> (x+y=w4316:i32)
                          n2192 = local read "csv作成表"() -> (w4312:string[][])
                          n2193 = Unbundle By Name(w4323) -> ("実測値(MAX)"=w4319:string, "実測値(MIN)"=w4320:string)
                          n2194 = Replace Array Subset(array=w4312, new element #1=w4319, index (row) #1=w4317, index (col) #1=w4318, new element #2=w4320, index (row) #2=w4317, index (col) #2=w4316) -> (w4314:string[][])
                          n2195 = Select(t=w4314, s=w4324, f=w4312) -> (s? t:f=w4315:string[][])
                          n2196 = local write "csv作成表"(w4315) -> ()
                        }
                        frame 3 {
                          w4335 = 2
                          # "B"
                          # "A"
                          # "csv作成の為表へクラスタ(実測値)書き込み"
                          # "⑤"
                          # "③"
                          # "④"
                          n2197 = local read "メインON/OFF_\n設定 4"() -> (w4346:T1)
                          n2198 = Unbundle By Name(w4346) -> ("使用ON/OFF"=w4342:bool)
                          n2199 = control-ref of="前回値転記用配列"() -> (w4340:refnum<vi>)
                          n2200 = local read "メイン設定_設定 4"() -> (w4347:T2)
                          n2201 = call "メイン_測定値配列_CSV転記サブ.vi"("メイン設定_設定入力"=w4347, "ループ反復数値入力"=w4344, "実測設定項目"=w4345, "使用ON/OFF"=w4342, "前回値転記用配列"=w4340) -> ("ループ反復数値出力"=w4343:i32, "メイン設定_設定出力"=w4341:T2)  [unwired: 5 in]
                          n2202 = local write "メイン設定_設定 4"(w4341) -> ()
                          n2203 = Add(x=5, y=w4343) -> (x+y=w4336:i32)
                          n2204 = Add(x=w4343, y=6) -> (x+y=w4334:i32)
                          n2205 = local read "csv作成表"() -> (w4330:string[][])
                          n2206 = Unbundle By Name(w4341) -> ("実測値(MAX)"=w4337:string, "実測値(MIN)"=w4338:string)
                          n2207 = Replace Array Subset(array=w4330, new element #1=w4337, index (row) #1=w4335, index (col) #1=w4336, new element #2=w4338, index (row) #2=w4335, index (col) #2=w4334) -> (w4332:string[][])
                          n2208 = Select(t=w4332, s=w4342, f=w4330) -> (s? t:f=w4333:string[][])
                          n2209 = local write "csv作成表"(w4333) -> ()
                        }
                        frame 4 {
                          w4353 = 2
                          # "B"
                          # "A"
                          # "csv作成の為表へクラスタ(実測値)書き込み"
                          # "⑤"
                          # "③"
                          # "④"
                          n2210 = local read "メインON/OFF_\n設定 5"() -> (w4364:T1)
                          n2211 = Unbundle By Name(w4364) -> ("使用ON/OFF"=w4360:bool)
                          n2212 = control-ref of="前回値転記用配列"() -> (w4358:refnum<vi>)
                          n2213 = local read "メイン設定_設定 5"() -> (w4365:T2)
                          n2214 = call "メイン_測定値配列_CSV転記サブ.vi"("メイン設定_設定入力"=w4365, "ループ反復数値入力"=w4362, "実測設定項目"=w4363, "使用ON/OFF"=w4360, "前回値転記用配列"=w4358) -> ("ループ反復数値出力"=w4361:i32, "メイン設定_設定出力"=w4359:T2)  [unwired: 5 in]
                          n2215 = local write "メイン設定_設定 5"(w4359) -> ()
                          n2216 = Add(x=6, y=w4361) -> (x+y=w4354:i32)
                          n2217 = Add(x=w4361, y=7) -> (x+y=w4352:i32)
                          n2218 = local read "csv作成表"() -> (w4348:string[][])
                          n2219 = Unbundle By Name(w4359) -> ("実測値(MAX)"=w4355:string, "実測値(MIN)"=w4356:string)
                          n2220 = Replace Array Subset(array=w4348, new element #1=w4355, index (row) #1=w4353, index (col) #1=w4354, new element #2=w4356, index (row) #2=w4353, index (col) #2=w4352) -> (w4350:string[][])
                          n2221 = Select(t=w4350, s=w4360, f=w4348) -> (s? t:f=w4351:string[][])
                          n2222 = local write "csv作成表"(w4351) -> ()
                        }
                        frame 5 {
                          w4371 = 2
                          # "B"
                          # "A"
                          # "csv作成の為表へクラスタ(実測値)書き込み"
                          # "⑤"
                          # "③"
                          # "④"
                          n2223 = local read "メインON/OFF_\n設定 6"() -> (w4382:T1)
                          n2224 = Unbundle By Name(w4382) -> ("使用ON/OFF"=w4378:bool)
                          n2225 = control-ref of="前回値転記用配列"() -> (w4376:refnum<vi>)
                          n2226 = local read "メイン設定_設定 6"() -> (w4383:T2)
                          n2227 = call "メイン_測定値配列_CSV転記サブ.vi"("メイン設定_設定入力"=w4383, "ループ反復数値入力"=w4380, "実測設定項目"=w4381, "使用ON/OFF"=w4378, "前回値転記用配列"=w4376) -> ("ループ反復数値出力"=w4379:i32, "メイン設定_設定出力"=w4377:T2)  [unwired: 5 in]
                          n2228 = local write "メイン設定_設定 6"(w4377) -> ()
                          n2229 = Add(x=7, y=w4379) -> (x+y=w4372:i32)
                          n2230 = Add(x=w4379, y=8) -> (x+y=w4370:i32)
                          n2231 = local read "csv作成表"() -> (w4366:string[][])
                          n2232 = Unbundle By Name(w4377) -> ("実測値(MAX)"=w4373:string, "実測値(MIN)"=w4374:string)
                          n2233 = Replace Array Subset(array=w4366, new element #1=w4373, index (row) #1=w4371, index (col) #1=w4372, new element #2=w4374, index (row) #2=w4371, index (col) #2=w4370) -> (w4368:string[][])
                          n2234 = Select(t=w4368, s=w4378, f=w4366) -> (s? t:f=w4369:string[][])
                          n2235 = local write "csv作成表"(w4369) -> ()
                        }
                        frame 6 {
                          w4389 = 2
                          # "B"
                          # "A"
                          # "csv作成の為表へクラスタ(実測値)書き込み"
                          # "⑤"
                          # "③"
                          # "④"
                          n2236 = local read "メインON/OFF_\n設定 7"() -> (w4400:T1)
                          n2237 = Unbundle By Name(w4400) -> ("使用ON/OFF"=w4396:bool)
                          n2238 = control-ref of="前回値転記用配列"() -> (w4394:refnum<vi>)
                          n2239 = local read "メイン設定_設定 7"() -> (w4401:T2)
                          n2240 = call "メイン_測定値配列_CSV転記サブ.vi"("メイン設定_設定入力"=w4401, "ループ反復数値入力"=w4398, "実測設定項目"=w4399, "使用ON/OFF"=w4396, "前回値転記用配列"=w4394) -> ("ループ反復数値出力"=w4397:i32, "メイン設定_設定出力"=w4395:T2)  [unwired: 5 in]
                          n2241 = local write "メイン設定_設定 7"(w4395) -> ()
                          n2242 = Add(x=8, y=w4397) -> (x+y=w4390:i32)
                          n2243 = Add(x=w4397, y=9) -> (x+y=w4388:i32)
                          n2244 = local read "csv作成表"() -> (w4384:string[][])
                          n2245 = Unbundle By Name(w4395) -> ("実測値(MAX)"=w4391:string, "実測値(MIN)"=w4392:string)
                          n2246 = Replace Array Subset(array=w4384, new element #1=w4391, index (row) #1=w4389, index (col) #1=w4390, new element #2=w4392, index (row) #2=w4389, index (col) #2=w4388) -> (w4386:string[][])
                          n2247 = Select(t=w4386, s=w4396, f=w4384) -> (s? t:f=w4387:string[][])
                          n2248 = local write "csv作成表"(w4387) -> ()
                        }
                        frame 7 {
                          w4407 = 2
                          # "B"
                          # "A"
                          # "csv作成の為表へクラスタ(実測値)書き込み"
                          # "⑤"
                          # "③"
                          # "④"
                          n2249 = local read "メインON/OFF_\n設定 8"() -> (w4418:T1)
                          n2250 = Unbundle By Name(w4418) -> ("使用ON/OFF"=w4414:bool)
                          n2251 = control-ref of="前回値転記用配列"() -> (w4412:refnum<vi>)
                          n2252 = local read "メイン設定_設定 8"() -> (w4419:T2)
                          n2253 = call "メイン_測定値配列_CSV転記サブ.vi"("メイン設定_設定入力"=w4419, "ループ反復数値入力"=w4416, "実測設定項目"=w4417, "使用ON/OFF"=w4414, "前回値転記用配列"=w4412) -> ("ループ反復数値出力"=w4415:i32, "メイン設定_設定出力"=w4413:T2)  [unwired: 5 in]
                          n2254 = local write "メイン設定_設定 8"(w4413) -> ()
                          n2255 = Add(x=9, y=w4415) -> (x+y=w4408:i32)
                          n2256 = Add(x=w4415, y=10) -> (x+y=w4406:i32)
                          n2257 = local read "csv作成表"() -> (w4402:string[][])
                          n2258 = Unbundle By Name(w4413) -> ("実測値(MAX)"=w4409:string, "実測値(MIN)"=w4410:string)
                          n2259 = Replace Array Subset(array=w4402, new element #1=w4409, index (row) #1=w4407, index (col) #1=w4408, new element #2=w4410, index (row) #2=w4407, index (col) #2=w4406) -> (w4404:string[][])
                          n2260 = Select(t=w4404, s=w4414, f=w4402) -> (s? t:f=w4405:string[][])
                          n2261 = local write "csv作成表"(w4405) -> ()
                        }
                        frame 8 {
                          w4425 = 2
                          # "B"
                          # "A"
                          # "csv作成の為表へクラスタ(実測値)書き込み"
                          # "⑤"
                          # "③"
                          # "④"
                          n2262 = local read "メインON/OFF_\n設定 9"() -> (w4436:T1)
                          n2263 = Unbundle By Name(w4436) -> ("使用ON/OFF"=w4432:bool)
                          n2264 = control-ref of="前回値転記用配列"() -> (w4430:refnum<vi>)
                          n2265 = local read "メイン設定_設定 9"() -> (w4437:T2)
                          n2266 = call "メイン_測定値配列_CSV転記サブ.vi"("メイン設定_設定入力"=w4437, "ループ反復数値入力"=w4434, "実測設定項目"=w4435, "使用ON/OFF"=w4432, "前回値転記用配列"=w4430) -> ("ループ反復数値出力"=w4433:i32, "メイン設定_設定出力"=w4431:T2)  [unwired: 5 in]
                          n2267 = local write "メイン設定_設定 9"(w4431) -> ()
                          n2268 = Add(x=10, y=w4433) -> (x+y=w4426:i32)
                          n2269 = Add(x=w4433, y=11) -> (x+y=w4424:i32)
                          n2270 = local read "csv作成表"() -> (w4420:string[][])
                          n2271 = Unbundle By Name(w4431) -> ("実測値(MAX)"=w4427:string, "実測値(MIN)"=w4428:string)
                          n2272 = Replace Array Subset(array=w4420, new element #1=w4427, index (row) #1=w4425, index (col) #1=w4426, new element #2=w4428, index (row) #2=w4425, index (col) #2=w4424) -> (w4422:string[][])
                          n2273 = Select(t=w4422, s=w4432, f=w4420) -> (s? t:f=w4423:string[][])
                          n2274 = local write "csv作成表"(w4423) -> ()
                        }
                        frame 9 {
                          w4443 = 2
                          # "B"
                          # "A"
                          # "csv作成の為表へクラスタ(実測値)書き込み"
                          # "⑤"
                          # "③"
                          # "④"
                          n2275 = local read "メインON/OFF_\n設定 10"() -> (w4454:T1)
                          n2276 = Unbundle By Name(w4454) -> ("使用ON/OFF"=w4450:bool)
                          n2277 = control-ref of="前回値転記用配列"() -> (w4448:refnum<vi>)
                          n2278 = local read "メイン設定_設定 10"() -> (w4455:T2)
                          n2279 = call "メイン_測定値配列_CSV転記サブ.vi"("メイン設定_設定入力"=w4455, "ループ反復数値入力"=w4452, "実測設定項目"=w4453, "使用ON/OFF"=w4450, "前回値転記用配列"=w4448) -> ("ループ反復数値出力"=w4451:i32, "メイン設定_設定出力"=w4449:T2)  [unwired: 5 in]
                          n2280 = local write "メイン設定_設定 10"(w4449) -> ()
                          n2281 = Add(x=11, y=w4451) -> (x+y=w4444:i32)
                          n2282 = Add(x=w4451, y=12) -> (x+y=w4442:i32)
                          n2283 = local read "csv作成表"() -> (w4438:string[][])
                          n2284 = Unbundle By Name(w4449) -> ("実測値(MAX)"=w4445:string, "実測値(MIN)"=w4446:string)
                          n2285 = Replace Array Subset(array=w4438, new element #1=w4445, index (row) #1=w4443, index (col) #1=w4444, new element #2=w4446, index (row) #2=w4443, index (col) #2=w4442) -> (w4440:string[][])
                          n2286 = Select(t=w4440, s=w4450, f=w4438) -> (s? t:f=w4441:string[][])
                          n2287 = local write "csv作成表"(w4441) -> ()
                        }
                        frame 10 {
                          w4461 = 2
                          # "B"
                          # "A"
                          # "csv作成の為表へクラスタ(実測値)書き込み"
                          # "⑤"
                          # "③"
                          # "④"
                          n2288 = local read "メインON/OFF_\n設定 11"() -> (w4472:T1)
                          n2289 = Unbundle By Name(w4472) -> ("使用ON/OFF"=w4468:bool)
                          n2290 = control-ref of="前回値転記用配列"() -> (w4466:refnum<vi>)
                          n2291 = local read "メイン設定_設定 11"() -> (w4473:T2)
                          n2292 = call "メイン_測定値配列_CSV転記サブ.vi"("メイン設定_設定入力"=w4473, "ループ反復数値入力"=w4470, "実測設定項目"=w4471, "使用ON/OFF"=w4468, "前回値転記用配列"=w4466) -> ("ループ反復数値出力"=w4469:i32, "メイン設定_設定出力"=w4467:T2)  [unwired: 5 in]
                          n2293 = local write "メイン設定_設定 11"(w4467) -> ()
                          n2294 = Add(x=12, y=w4469) -> (x+y=w4462:i32)
